vi "PH_SSAC._PC Cam linked.vi"(0 "i ref in":refnum<vi>, 2 "cam not linked?":bool, 5 "error IO":errorcluster) -> (14 "i ref out":refnum<vi>, 19 "error out":errorcluster)   [LabVIEW 2014, in "PH_SSAC.lvlib"]
doc: "This is a certain proc case."
uses:
  PH_SSAC.lvlib
  PH_Common/PH_Common.lvlib
  PH_Img_BaseClass/PH_Img_BaseClass.lvlib
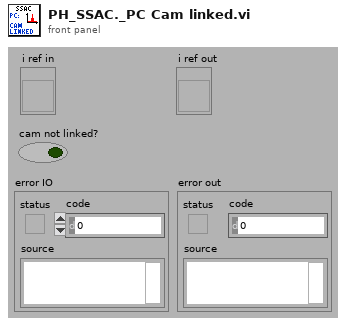
[diagram p1: front panel]
types:
  T1 = enum8{"Enabled", "Disabled", "Disabled and Grayed Out"}
  T2 = typedef "PH_Img_BaseClass.lvlib/PH_Img_BaseClass.i attribute.ctl" = cluster{"GUI Refs":T3, "Timeout Image [ms]":i32, "Default Periodic Period [ms]":i32, "Camera":cluster{"Instancename":string, "Notifier":refnum<notifier>}, "Palette":T4, "Cam Settings":cluster{"Cam ID":string, "Gain":dbl, "Brightness":dbl, "Shutter":dbl, "Cam Info Failure":bool, "Mode":i32}}
  T3 = typedef "PH_Img_BaseClass.lvlib/PH_Img_BaseClass.GUI Refs.ctl" = cluster{"Timeout":refnum<vi>, "Image":refnum<vi>, "Palette":refnum<vi>, "Timeout Set":refnum<vi>}
  T4 = typedef "PH_Img_BaseClass.lvlib/PH_Img_BaseClass.Palette.ctl" = i32
  T5 = typedef "PH_SSAC.lvlib/PH_SSAC.i attribute.ctl" = cluster{"GUI Refs":cluster{"Delete":refnum<vi>, "Global On":refnum<vi>, "Cam Source":refnum<vi>, "Frame Main Signal":refnum<vi>, "Frame Background":refnum<vi>, "dt (Gauss smooth)":refnum<vi>, "Calibration Factor":refnum<vi>, "Background acquire":refnum<vi>, "Threshold":refnum<vi>, "Time evolution of mean pulse duration":refnum<vi>, "Mean Pulse Duration":refnum<vi>, "Main signal":refnum<vi>, "Current Pulse Duration":refnum<vi>, "Processed":refnum<vi>, "Saturation":refnum<vi>, "# for Average":refnum<vi>, "Position":refnum<vi>, "BG Status":refnum<vi>, "Save BG data":refnum<vi>, "Read BG Data":refnum<vi>, "Background Calibration Data":refnum<vi>}, "Images":cluster{"OP Image":T6, "GUI Image":T6, "PSDB Image":T6}, "Global On?":bool, "Frame Main":cluster{"x":u32, "dx":u32, "y":u32, "dy":u32}, "Frame Background":cluster{"x":u32, "dx":u32, "y":u32, "dy":u32}, "dt [fs]":dbl, "Calibration Factor [fs/pixel]":dbl, "Threshold":dbl, "Time evolution of mean pulse duration [fs]":dbl[], "Main Signal":cluster{"Time for Main":dbl[], "Signal":dbl[]}, "Processed":bool, "Current Pulse Duration [fs]":dbl, "# for Average":i32, "Position":i32, "Pulse Durations [fs]":dbl[], "BG":cluster{"Acquire?":bool, "Background Calibration Data":T7, "Save Data":bool}}
  T6 = typedef "IMAQ Image.ctl" = refnum<image>
  T7 = typedef "PH_SSAC.lvlib/PH_SSAC.Background Data.ctl" = cluster{"Date":string, "Time":string, "Frame Main":cluster{"x":u32, "dx":u32, "y":u32, "dy":u32}, "dt [fs]":dbl, "Calibration Factor [fs/pixel]":dbl, "Signal":dbl[], "Frame Background":cluster{"x":u32, "dx":u32, "y":u32, "dy":u32}}
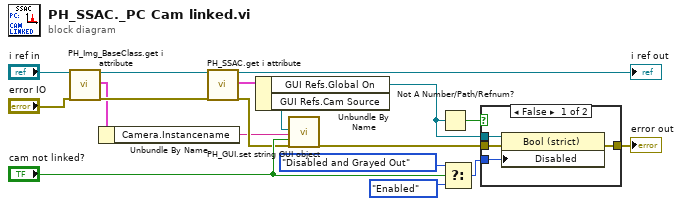
[diagram p0: block diagram]
diagram:
  n1 = call "PH_Img_BaseClass.get i attribute.vi"("i ref in"="i ref in", "error in (no error)"="error IO") -> ("i ref out"=w5:refnum<vi>, "i attribute"=w4:T2, "error out"=w7:errorcluster)  [unwired: 15 in]
  n2 = Unbundle By Name(w4) -> ("Camera.Instancename"=w3:string)
  n3 = call "PH_SSAC.get i attribute.vi"("i ref in"=w5, "error in (no error)"=w7) -> ("i ref out"=→"i ref out":refnum<vi>, "i attribute"=w17:T5, "error out"=w16:errorcluster)  [unwired: 15 in]
  n4 = Unbundle By Name(w17) -> ("GUI Refs.Global On"=w11:refnum<vi>, "GUI Refs.Cam Source"=w14:refnum<vi>)
  n5 = call "PH_GUI.set string GUI object.vi"("GUI object Ref"=w14, "Text"=w3, "Blinking? (false)"="cam not linked?", "error in"=w16) -> ("error out"=w13:errorcluster)  [unwired: 15 in]
  n6 = Not A Number/Path/Refnum?(number/path/refnum=w11) -> (NaN/Path/Refnum?=w10:bool)
  n7 = Select(t=T1."Disabled and Grayed Out" ("Disabled"), s="cam not linked?", f=T1."Enabled" ("Disabled")) -> (s? t:f=w12:T1)
  n8 = case shown="False" w10 {
    tunnel: w13 -> [w22 w23]
    tunnel: [w21 w23] -> w8
    tunnel: w11 -> [w20 _]
    tunnel: w12 -> [w19 _]
    frame False {
      n9 = property class="Bool (strict)"(reference=w20, error in=w22, "Disabled"=w19) -> (error out=w21:errorcluster)  [unwired: 1 out]
    }
    frame True {
    }
  }
  "error out" <- w8
